vi "Day - 12 Hot Springs.vi"() -> ()   [LabVIEW 2020, in "AoC 2023.lvlib"]
uses:
  AoC 2023.lvlib
panel:
  in  "Tab Control":enum32{"Debug - I/p Data", ""}(tab)
  out "Input":cluster{"String":string, i32[]}[](array[cluster])
  out "GRID":string[][](array[string])
  in  "TIMEOUT":i32
  out "Puzzle Part-2 Answer":string
  out "Puzzle Answer":string
  in  "Puzzle Inputs":string[](array[string])=["???.### 1,1,3\n.??..??...?##. 1,1,3\n?#?#?#?#?#?#?#? 1,3,1,6\n????.#...#... 4,1,1\n????.######..#####. 1,6,5\n?###???????? 3,2,1"]
  # "Enter the Puzzle Input and run the VI"
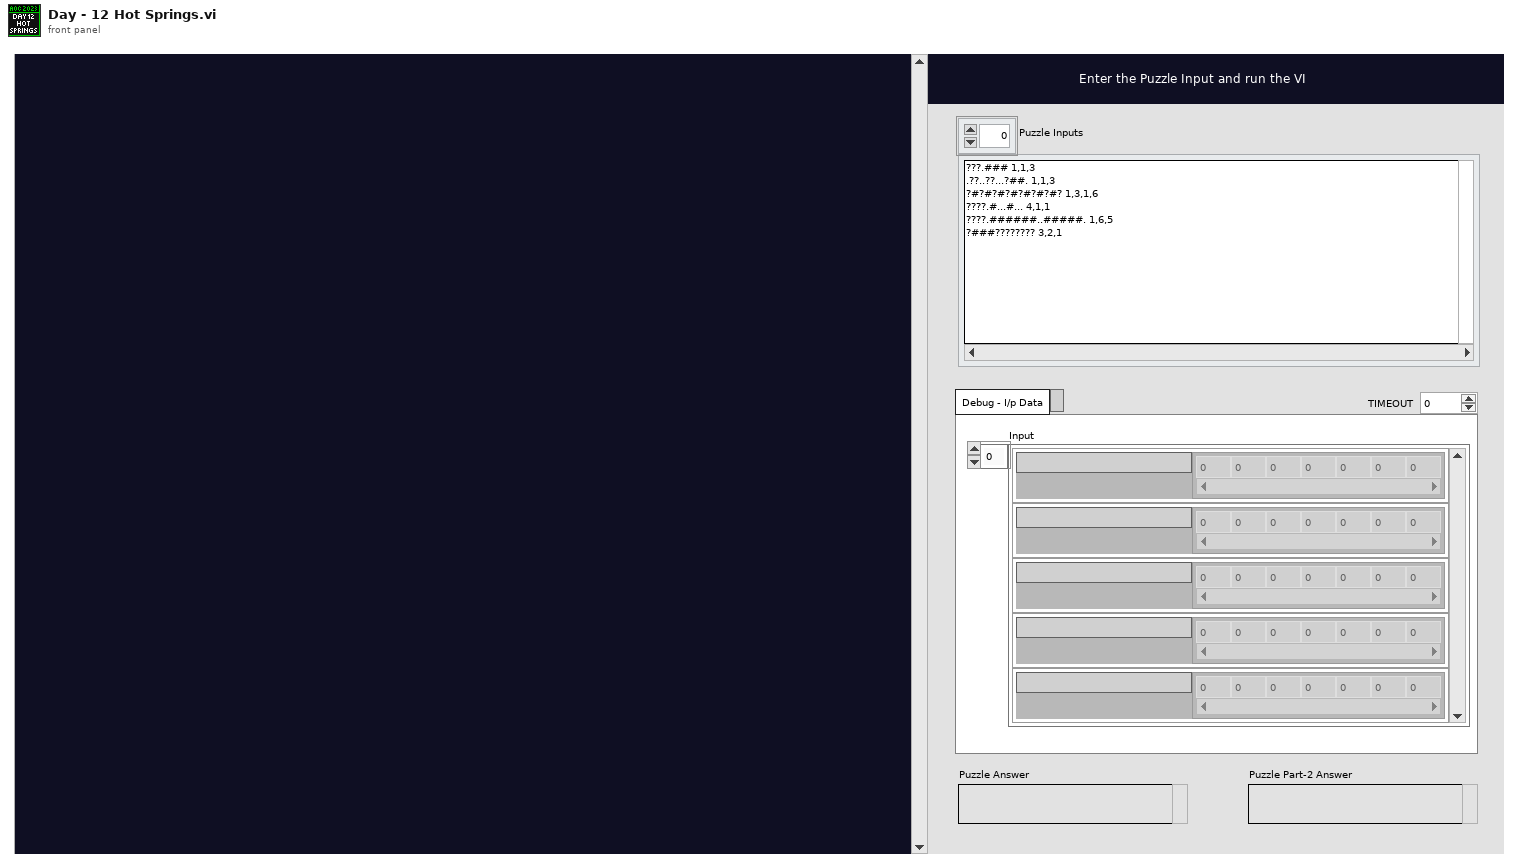
[diagram p1: front panel]
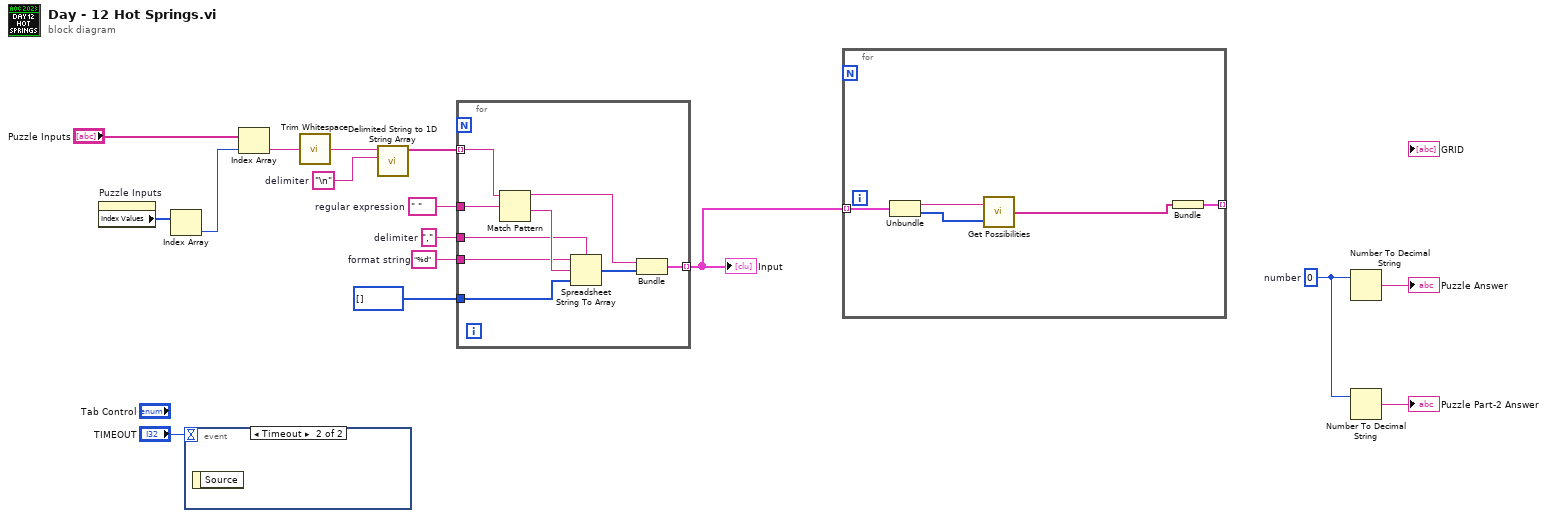
[diagram p0: block diagram]
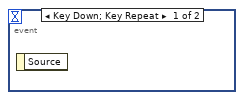
[diagram p2: hidden frame]
diagram:
  w2 = ","  # delimiter
  w4 = "%d"  # format string
  w5 = " "  # regular expression
  w7 = 0  # number
  w14 = "\n"  # delimiter
  n1 = property on="Puzzle Inputs" class="Arr (strict)"() -> ("Index Values"=w10:u32[])  [unwired: 2 in, 2 out]
  n2 = Index Array(array=w10) -> (element=w9:u32)  [unwired: 1 in]
  n3 = event shown="[1] Timeout" {
    selector: _ -> [_ _]
    dyn-events: _ -> [_ _]
    timeout: "TIMEOUT" -> [_ _]
    event Key Down; Key Repeat {
      n4 = event-data() -> ()  [unwired: 1 in, 1 out]
    }
    event Timeout {
      n5 = event-data() -> ()  [unwired: 1 in, 1 out]
    }
  }
  n6 = Index Array(array="Puzzle Inputs", index=w9) -> (element=w11:string)
  n7 = call <vilib>:"Trim Whitespace.vi"("string"=w11) -> ("trimmed string"=w13:string)  [unwired: 1 in]
  n8 = call <vilib>:"Delimited String to 1D String Array.vi"("delimiter"=w14, "delimited string"=w13) -> ("string array"=w6:string[])  [unwired: 9 in]
  n9 = for {
    tunnel: w6 -> [w25] mode=indexing
    tunnel: w5 -> [w24]
    tunnel: w4 -> [w22]
    tunnel: i32[] [] -> [w21]
    tunnel: [w18] -> w1 mode=indexing
    tunnel: w2 -> [w17]
    n10 = Match Pattern(string=w25, regular expression=w24) -> (before substring=w20:string, after substring=w23:string)  [unwired: 1 in, 2 out]
    n11 = Spreadsheet String To Array(delimiter (Tab)=w17, format string=w22, spreadsheet string=w23, array type (2D Dbl)=w21) -> (array=w19:i32[])
    n12 = Bundle("String"=w20, w19) -> (w18:cluster{"String":string, i32[]})  [unwired: 1 in]
  }
  "Input" <- w1
  n13 = for {
    tunnel: w1 -> [w28] mode=indexing
    tunnel: [w29] -> _ mode=indexing
    n14 = Unbundle(w28) -> ("String"=w26:string, w27:i32[])
    n15 = call "Get Possibilities.vi"("Damaged Springs"=w27, "Spring Record"=w26) -> ("Possible Spring Records"=w30:string[])
    n16 = Bundle("Possible Spring Records"=w30) -> (w29:cluster{"Possible Spring Records":string[]})  [unwired: 1 in]
  }
  n17 = Number To Decimal String(number=w7) -> (decimal integer string=→"Puzzle Answer":string)  [unwired: 1 in]
  n18 = Number To Decimal String(number=w7) -> (decimal integer string=→"Puzzle Part-2 Answer":string)  [unwired: 1 in]
